vi "Read Marker (Delta Marker).vi"(0 "VISA resource name":refnum<visa-resource-name>, 5 "Marker (0:Marker 1)":i32(ring) items=["Marker 1", "Marker 2", "Marker 3", "Marker 4", "Marker 5", "Marker 6", "Marker 7", "Marker 8", "Marker 9", "Marker 10"], 11 "error in (no error)":errorcluster) -> (4 "VISA resource name out":refnum<visa-resource-name>, 6 "Delta Marker Response":dbl format="%.3f", 15 "error out":errorcluster)   [LabVIEW 2023, in "Anritsu Signal Analyzer Series.lvlib"]
doc: "Queries the marker level in relative value."
uses:
  Anritsu Signal Analyzer Series.lvlib
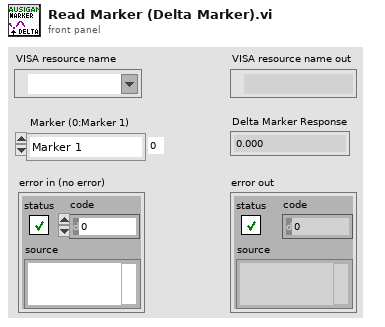
[diagram p1: front panel]
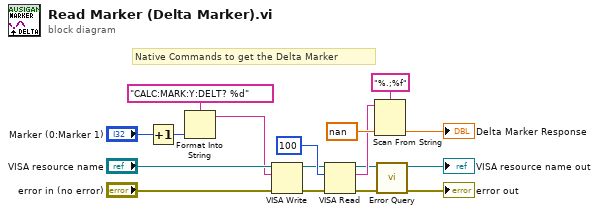
[diagram p0: block diagram]
diagram:
  # "Native Commands to get the Delta Marker"
  n1 = Increment(x="Marker (0:Marker 1)") -> (x+1=w2:i32)
  n2 = Format Into String(format string="CALC:MARK:Y:DELT? %d" ("_Command"), w2) -> (resulting string=w3:string)  [unwired: 2 in, 1 out]
  n3 = VISA Write(VISA resource name="VISA resource name", write buffer=w3, error in (no error)="error in (no error)") -> (VISA resource name out=w7:refnum<visa-resource-name>, error out=w8:errorcluster)  [unwired: 1 out]
  n4 = VISA Read(VISA resource name=w7, byte count=u32 100 ("byte count (0)"), error in (no error)=w8) -> (VISA resource name out=w5:refnum<visa-resource-name>, read buffer=w6:string, error out=w4:errorcluster)  [unwired: 1 out]
  n5 = Scan From String(format string="%.;%f" ("Format String"), input string=w6, default 1=nan ("_Default")) -> (output 1=→"Delta Marker Response":dbl)  [unwired: 2 in, 3 out]
  n6 = call "Error Query.vi"("error in (no error)"=w4, "VISA resource name"=w5) -> ("error out"=→"error out":errorcluster, "VISA resource name out"=→"VISA resource name out":refnum<visa-resource-name>)  [unwired: 6 in, 2 out]
